vi "GenerateDictionaryFromVIs.vi"(7 "VIs in":refnum<vi>[](array[refnum]), 8 "error in (no error)":errorcluster, 9 "Additional Languages [English]":string[](array[string])=["English"], 10 "Current VI Language (English)":string="English", 11 "Fonts []":T2[](array[typedef])) -> (0 "error out":errorcluster, 3 "Localization":T1)   [LabVIEW 2017, in "JKI Simple Localization.lvlib"]
uses:
  API/JKI Simple Localization.lvlib
  Definitions/Private/FontCluster.ctl
  Definitions/Dictionary--Cluster.ctl
  Definitions/Private/Phrase Dictionary.ctl
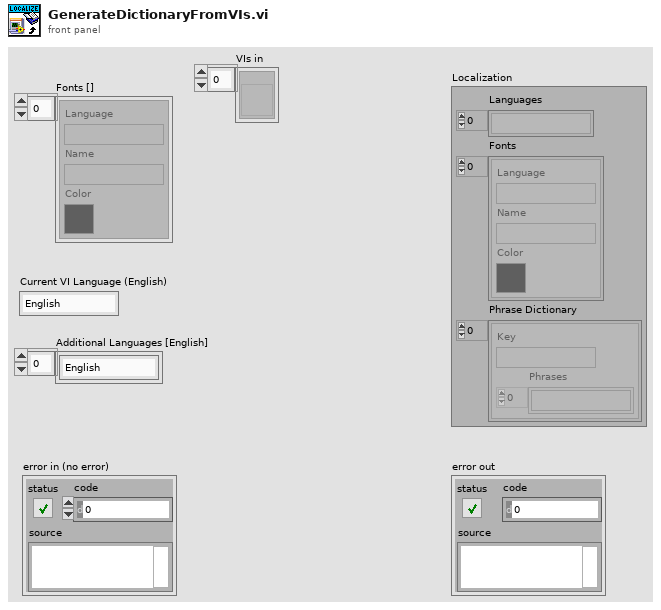
[diagram p1: front panel]
types:
  T1 = typedef "JKI Simple Localization.lvlib/Dictionary--Cluster.ctl" = cluster{"Languages":string[], "Fonts":T2[], "Phrase Dictionary":T3[]}
  T2 = typedef "JKI Simple Localization.lvlib/FontCluster.ctl" = cluster{"Language":string, "Name":string, "Color":u32}
  T3 = typedef "JKI Simple Localization.lvlib/Phrase Dictionary.ctl" = cluster{"Key":string, "Phrases":string[]}
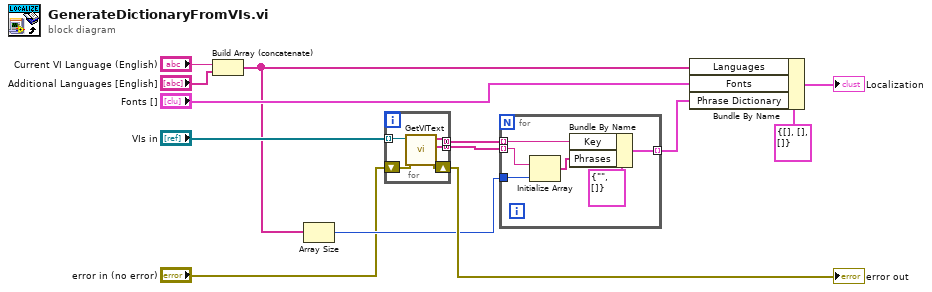
[diagram p0: block diagram]
diagram:
  n1 = Build Array (concatenate)("Current VI Language (English)", "Additional Languages [English]") -> (w1:string[])
  n2 = Array Size(array=w1) -> (size(s)=w11:i32)
  n3 = for {
    tunnel: "VIs in" -> [w18] mode=indexing
    tunnel: [w17] -> w7 mode=concatenating
    tunnel: [w16] -> w6 mode=concatenating
    shift-right: [w15] -> w13
    shift-left: "error in (no error)" -> [w14]
    n4 = call "GetVIText.vi"("error in (no error)"=w14, "VI"=w18) -> ("error out"=w15:errorcluster, "Control Text"=w17:string[], "Control Keys"=w16:string[])  [unwired: 7 in]
  }
  "error out" <- w13
  n5 = for {
    tunnel: w6 -> [w23] mode=indexing
    tunnel: w7 -> [w21] mode=indexing
    tunnel: w11 -> [w22]
    tunnel: [w19] -> w5 mode=indexing
    n6 = Initialize Array(w21, w22) -> (w20:string[])
    n7 = Bundle By Name(cluster=T3 {"Key"="", "Phrases"=[]} ("Phrase Dictionary"), "Key"=w23, "Phrases"=w20) -> (w19:T3)
  }
  n8 = Bundle By Name(cluster=T1 {"Languages"=[], "Fonts"=[], "Phrase Dictionary"=[]} ("Localization"), "Languages"=w1, "Fonts"="Fonts []", "Phrase Dictionary"=w5) -> (→"Localization":T1)
